vi "Set Reentrancy Type.vi"() -> ()   [LabVIEW 2015]
doc: "Parses <b>Search Path</b> for <b>File Type</b> and sets the \"Separate compiled code from source file\" option. Saves all modified files."
panel:
  in  "Reentrancy Type":T1(ring)
  out "Updated":u32
  out "Slide":u16(slide) caption="12/12" scale=-1.0..12.0
  out "error out":errorcluster
  out "All Files in Dir":path[](array[path])
  out "Array":errorcluster[](array[cluster])
  in  "Search Path":path
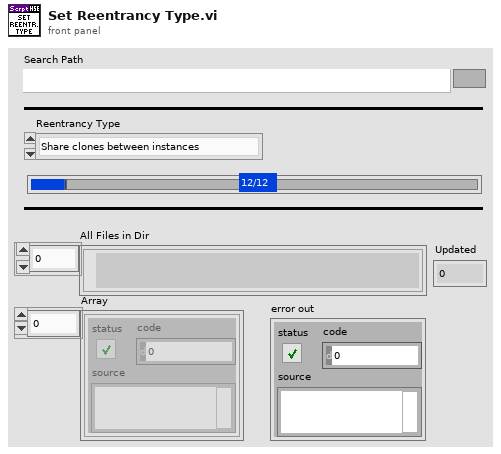
[diagram p1: front panel]
types:
  T1 = enum16{"Share clones between instances", "Preallocate clone for each instance"}
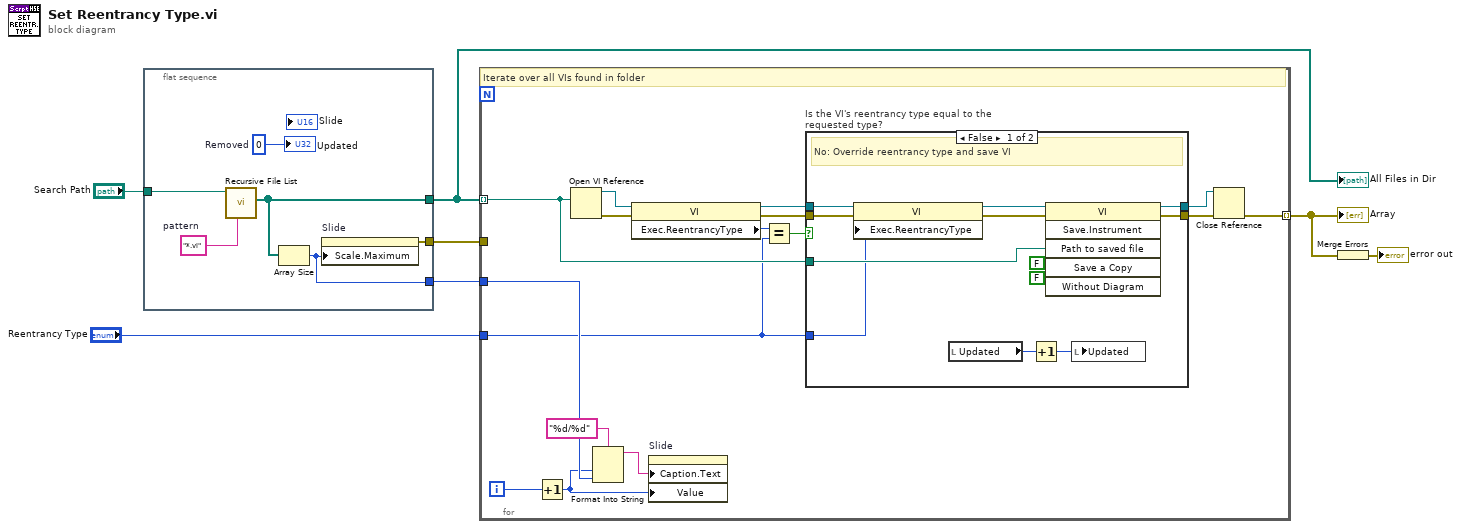
[diagram p0: block diagram]
diagram:
  n1 = flat-sequence {
    tunnel: "Search Path" -> [w13]
    tunnel: [w12] -> w4
    tunnel: [w11] -> w3
    tunnel: [w10] -> w2
    frame #0 {
      w8 = "*.vi"  # pattern
      w9 = u32 0  # Removed
      n2 = call <vilib>:"Recursive File List.vi"("pattern"=w8, "Folder Path"=w13) -> ("All Files in Dir"=w12:path[])  [unwired: 5 in, 4 out]
      n3 = Array Size(array=w12) -> (size(s)=w10:i32)
      n4 = property on="Slide" class="Slide (strict)"("Scale.Maximum"=w10) -> (error out=w11:errorcluster)  [unwired: 2 in, 1 out]
      "Updated" <- w9
    }
  }
  n5 = for {
    tunnel: w4 -> [w23] mode=indexing
    tunnel: [w29] -> w6 mode=indexing
    tunnel: w3 -> [_]
    tunnel: w2 -> [w27]
    tunnel: "Reentrancy Type" -> [w14]
    i -> [w28]
    # "Iterate over all VIs found in folder"
    n6 = Increment(x=w28) -> (x+1=w24:i32)
    n7 = Open VI Reference(vi path=w23) -> (vi reference=w20:refnum<vi>, error out=w19:errorcluster)  [unwired: 5 in]
    n8 = Format Into String(format string="%d/%d", w24, w27) -> (resulting string=w25:string)  [unwired: 2 in, 1 out]
    n9 = property class="VI"(reference=w20, error in=w19) -> (reference out=w18:refnum<vi>, error out=w17:errorcluster, "Exec.ReentrancyType"=w16:T1)
    n10 = property on="Slide" class="Slide (strict)"("Caption.Text"=w25, "Value"=w24) -> ()  [unwired: 2 in, 2 out]
    n11 = Equal?(x=w16, y=w14) -> (x = y?=w15:bool)
    n12 = case "Is the VI's reentrancy type equal to the requested type?" shown="False" w15 {
      tunnel: [w41 w43] -> w22
      tunnel: [w40 w42] -> w21
      tunnel: w23 -> [w35 _]
      tunnel: w18 -> [w34 w42]
      tunnel: w17 -> [w33 w43]
      tunnel: w14 -> [w30 _]
      frame False {
        # "No: Override reentrancy type and save VI"
        n13 = property class="VI"(reference=w34, error in=w33, "Exec.ReentrancyType"=w30) -> (reference out=w37:refnum<vi>, error out=w36:errorcluster)
        n14 = local read "Updated"() -> (w32:u32)
        n15 = Increment(x=w32) -> (x+1=w31:u32)
        n16 = invoke class="VI" method="Save.Instrument"(reference=w37, error in=w36, "Path to saved file"=w35, "Save a Copy"=FALSE, "Without Diagram"=FALSE) -> (reference out=w40:refnum<vi>, error out=w41:errorcluster)  [unwired: 1 in, 4 out]
        n17 = local write "Updated"(w31) -> ()
      }
      frame True {
        # "Yes: Do nothing"
      }
    }
    n18 = Close Reference(reference=w21, error in (no error)=w22) -> (error out=w29:errorcluster)
  }
  "Array" <- w6
  n19 = Merge Errors(w6) -> (→"error out":errorcluster)
  "All Files in Dir" <- w4
